vi "Close.vi"(8 "error in":errorcluster, 11 "CR5 in":refnum<class "CR5.lvclass">) -> (0 "error out":errorcluster, 3 "CR5 out":refnum<class "CR5.lvclass">)   [LabVIEW 2015, in "CR5.lvclass"]
uses:
  CR5.lvclass
  Reusable/Session APIs/Serial/Serial Session.lvclass
  CR5.lvclass/CR5.ctl
  Configurable Device/Configurable Device.lvclass
  <userlib>/_Session Fwk/Session - Root.lvclass
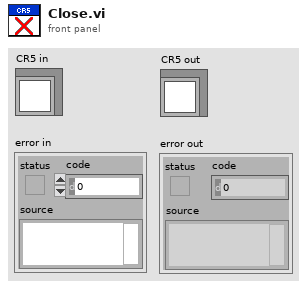
[diagram p1: front panel]
types:
  T1 = typedef "Session - Root.lvclass/Session Handle.ctl" = refnum<data-value>
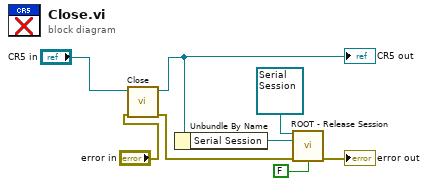
[diagram p0: block diagram]
diagram:
  n1 = call-parent "Close.vi"("error in"="error in", "Cfg Dev in"="CR5 in") -> ("error out"=w1:errorcluster, "Cfg Dev out"=w3:refnum<class "CR5.lvclass">)  [unwired: 8 in]
  "CR5 out" <- w3
  n2 = Unbundle By Name(w3) -> ("Serial Session"=w8:T1)
  n3 = call <userlib>:"ROOT - Release Session.vi"("OBJ - Session in"=refnum<class "Serial Session.lvclass"> refnum ("Serial Session"), "Session Handle in"=w8, "error in (no error)"=w1, "force destroy? (F)"=FALSE) -> ("error out"=→"error out":errorcluster)  [unwired: 10 in, 1 out]
